vi "CS_schleife_AMI.vi"() -> ()   [LabVIEW 2016]
uses:
  Equipment/Oxford Software/Oxsoft/RAMP.LLB/RampHState.ctl
  Equipment/Oxford Software/Oxsoft/RAMP.LLB/RampTState.ctl
  Global/Global Variables/global.vi
  Global/Global Variables/Data_Display_global.vi
  Instrument_Setup.vi
panel:
  in  "Ramp Parameters":T1 {"Sweep rate" format="%.2f"; "Field required:" format="%.2f"}
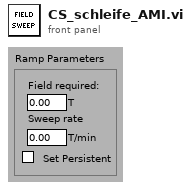
[diagram p1: front panel]
types:
  T1 = cluster{"Field required:":dbl[unit], "Sweep rate":dbl[unit], "Set Persistent":bool}
  T2 = typedef "RampHState.ctl" = enum16{"START", "RUN"}
  T3 = typedef "RampTState.ctl" = enum16{"START", "RUN"}
  T4 = typedef "PSIO.ctl" = cluster{"Address":T5, "Version":enum16{"PS", "IPS"}}
  T5 = typedef "OxfordAddress.ctl" = cluster{"Com Port":i32, "ISOBUS Address":i32, "GPIB Address":i16, "Communication":enum16{"RS232", "ISOBUS", "GPIB", "Gateway"}}
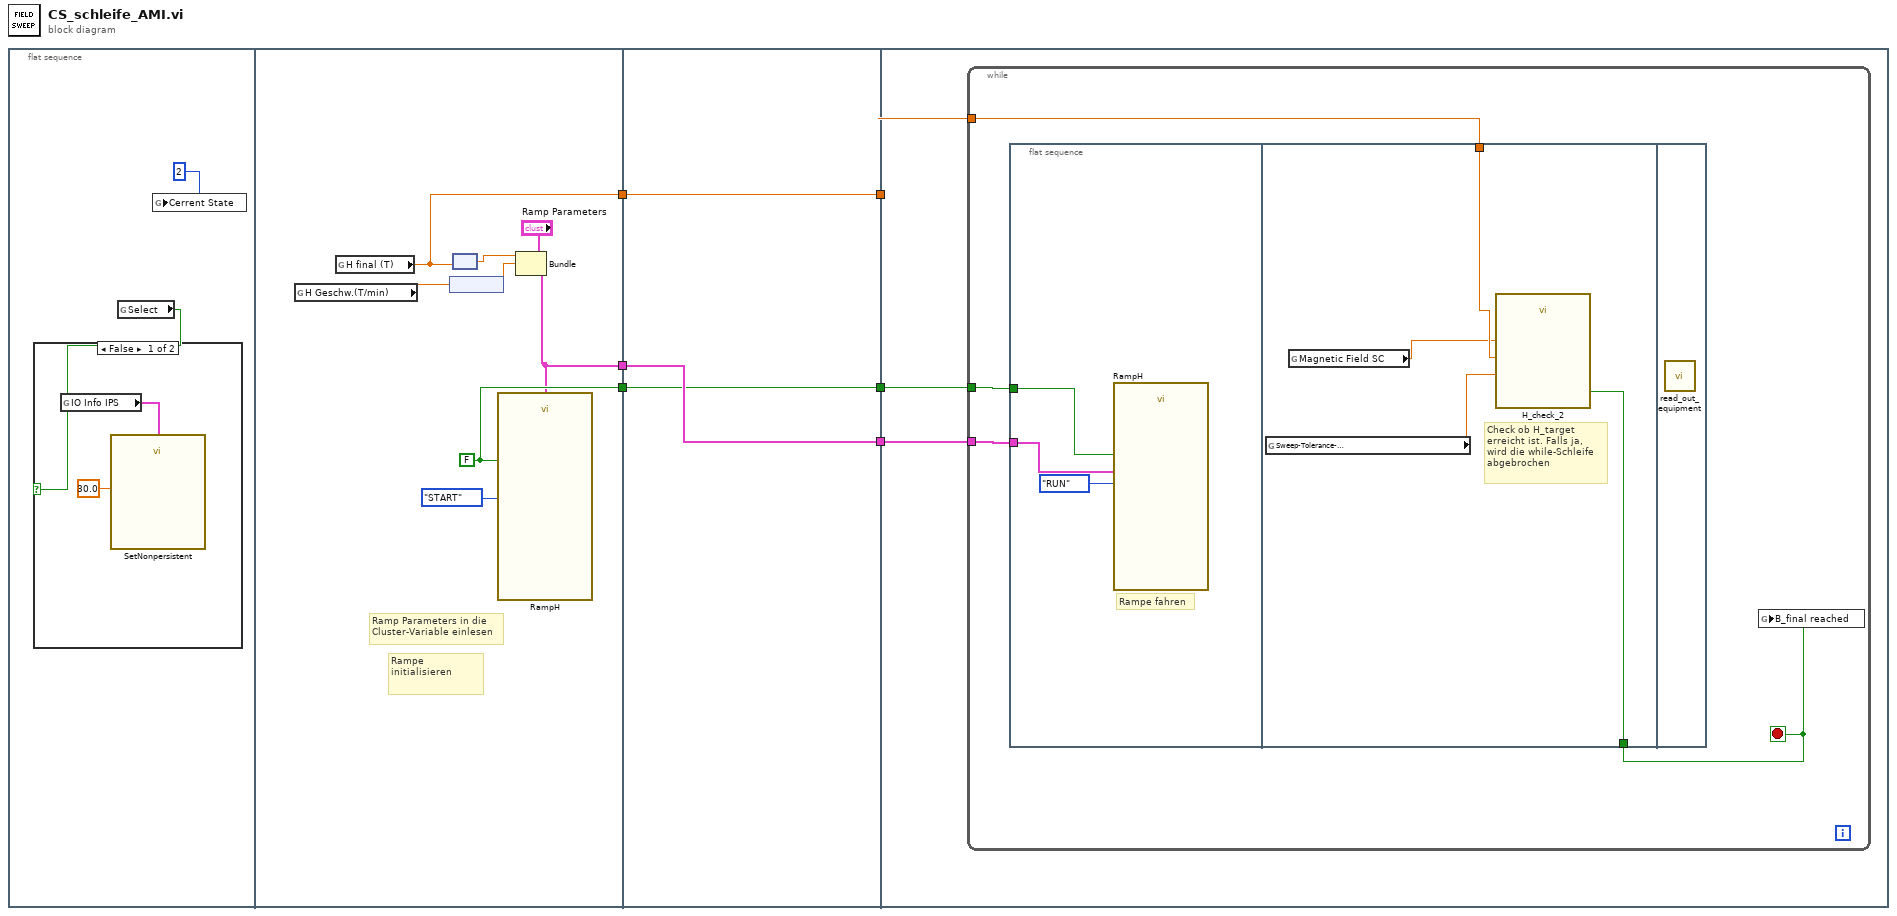
[diagram p0: block diagram]
diagram:
  n1 = flat-sequence {
    tunnel: [w13] -> w6
    tunnel: [w12] -> w4
    tunnel: [w11] -> w3
    tunnel: w6 -> [w21]
    tunnel: [w21] -> w5
    tunnel: w4 -> [w19]
    tunnel: w3 -> [w20]
    tunnel: [w20] -> w2
    tunnel: [w19] -> w1
    tunnel: w5 -> [w24]
    tunnel: w2 -> [w23]
    tunnel: w1 -> [w22]
    frame #0 {
      n2 = global read "Data_Display_global.vi" "Select"() -> (w7:bool)
      n3 = case shown="False" w7 {
        frame False {
          n4 = global read "Instrument_Setup.vi" "IO Info IPS"() -> (w10:T4)
          n5 = call "SetNonpersistent.vi"("Switch Heater Dwell Time"=dbl[unit] 30.0, "IO Info"=w10) -> ()  [unwired: 2 out]
        }
        frame True {
        }
      }
      n6 = global write "global.vi" "Cerrent State"(2) -> ()
    }
    frame #1 {
      w12 = FALSE ("JustReadTemperature")
      # "Rampe initialisieren"
      # "Ramp Parameters in die \nCluster-Variable einlesen"
      n7 = global read "global.vi" "H Geschw.(T/min)"() -> (w18:dbl)
      n8 = global read "global.vi" "H final (T)"() -> (w13:dbl)
      n9 = node(w18) -> (w14:dbl[unit])
      n10 = node(w13) -> (w15:dbl[unit])
      n11 = Bundle(cluster="Ramp Parameters", "Field required:"=w15, "Sweep rate"=w14) -> (w11:T1)  [unwired: 1 in]
      n12 = call "RampH.vi"("Ramp Parameters"=w11, "JustReadField"=w12, "RampHState"=RampHState."START") -> ()  [unwired: 4 in, 5 out]
    }
    frame #2 {
    }
    frame #3 {
      n13 = while {
        tunnel: w24 -> [w27]
        tunnel: w23 -> [w26]
        tunnel: w22 -> [w25]
        stop <- w28 stop-if-true
        n14 = flat-sequence {
          tunnel: w26 -> [w30]
          tunnel: w25 -> [w29]
          tunnel: [w35] -> w28
          tunnel: w27 -> [w33]
          frame #0 {
            # "Rampe fahren"
            n15 = call "RampH.vi"("Ramp Parameters"=w30, "JustReadField"=w29, "RampHState"=RampTState."RUN" ("RampTState")) -> ()  [unwired: 4 in, 5 out]
          }
          frame #1 {
            # "Check ob H_target\nerreicht ist. Falls ja,\nwird die while-Schleife\nabgebrochen"
            n16 = global read "Instrument_Setup.vi" "Sweep-Tolerance-\nMagnetic-Field"() -> (w34:dbl)
            n17 = global read "Data_Display_global.vi" "Magnetic Field SC"() -> (w32:dbl)
            n18 = call "H_check_2.vi"("Sweep\nTolerance %"=w34, "H_in"=w32, "H_target (K)"=w33) -> ("= H target"=w35:bool)  [unwired: 8 in]
          }
          frame #2 {
            n19 = call "read_out_equipment.vi"() -> ()  [unwired: 1 in]
          }
        }
        n20 = global write "Data_Display_global.vi" "B_final reached"(w28) -> ()
      }
    }
  }
